vi "main.vi"() -> ()   [LabVIEW 2014]
uses:
  mainVIs/wczytajDaneDoRuchuVIs/Akcje_wczytywania_danych_do_ruchu.ctl
  mainVIs/wykonajRuchVIs/parametryKomorVIs/WyborKomory.ctl
  mainVIs/AkcjaGFV.ctl
  mainVIs/Stan_glowny.ctl
  <vilib>/MakerHub/LINX/Public/Utilities/Open Local.vi
  <vilib>/MakerHub/LINX/LMH-LINX.lvlib
panel:
  out "Pomiar":bool
  out "Czujnik":bool
  in  "Stop":bool
  in  "Dӣ":bool
  in  "GÓRA":bool
  in  "LEWO":bool
  in  "PRAWO":bool
  in  "Praca ręczna":bool
  in  "Start":bool
  out "Działanie ramienia":bool
  out "Góra":bool
  out "Dół":bool
  out "Prawo":bool
  out "Lewo":bool
  # "Praca ręczna"
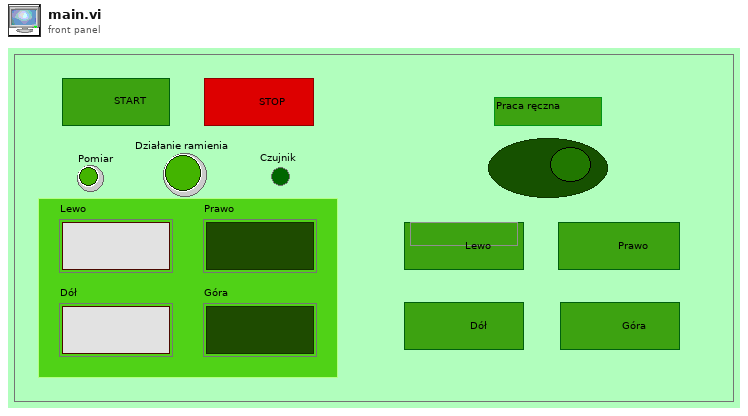
[diagram p1: front panel]
types:
  T1 = typedef "WyborKomory.ctl" = enum16{"NADAWCZA", "ODBIORCZA"}
  T2 = typedef "Akcje_wczytywania_danych_do_ruchu.ctl" = enum16{"Init", "Reset ramienia", "Przygotuj listę", "Sprawdź", "Koniec"}
  T3 = typedef "Stan_glowny.ctl" = enum16{"Oczekiwanie", "Init", "Działanie"}
  T4 = typedef "AkcjaGFV.ctl" = enum16{"Czytaj", "Zapisz", "Reset"}
  T5 = typedef "LMH-LINX.lvlib/LINX Ref.ctl" = cluster{"IO":T6, "Interface":T7, "LINX Device Config":T8}
  T6 = typedef "LMH-LINX.lvlib/Platform.ctl" = enum16{"Remote", "Local"}
  T7 = typedef "LMH-LINX.lvlib/Interface.ctl" = enum16{"Serial", "TCP"}
  T8 = typedef "LMH-LINX.lvlib/Device.lvlib/LINX Device Config.ctl" = cluster{"Interface":T7, "COM Port":refnum<visa-resource-name>, "TCP Configuration":T9, "Device Family":u8, "Device ID":u8, "Device Name":string, "TCP Ref":refnum<k5>, "Channels":T10}
  T9 = typedef "LMH-LINX.lvlib/Device.lvlib/TCP Config.ctl" = cluster{"IP Address":string, "Port":u16}
  T10 = typedef "LMH-LINX.lvlib/Channels.ctl" = cluster{"DI":u8[], "DO":u8[], "AI":u8[], "AO":u8[], "PWM":u8[], "QE":u8[], "UART":u8[], "I2C 2":u8[], "SPI":u8[], "CAN":u8[], "Servo":u8[], "AI Ref (V)":dbl, "AI Resolution (Bits)":u8, "AO Ref (V)":dbl, "AO Resolution (Bits)":u8}
  T11 = typedef "Przyciski_zbior.ctl" = cluster{"LEWO":bool, "PRAWO":bool, "GÓRA":bool, "Dӣ":bool, "Stop":bool, "Start":bool, "Praca ręczna":bool}
  T12 = typedef "Diody_zbior.ctl" = cluster{"Lewo":bool, "Prawo":bool, "Góra":bool, "Dół":bool, "Działanie":bool, "Czujnik":bool, "Pomiar":bool}
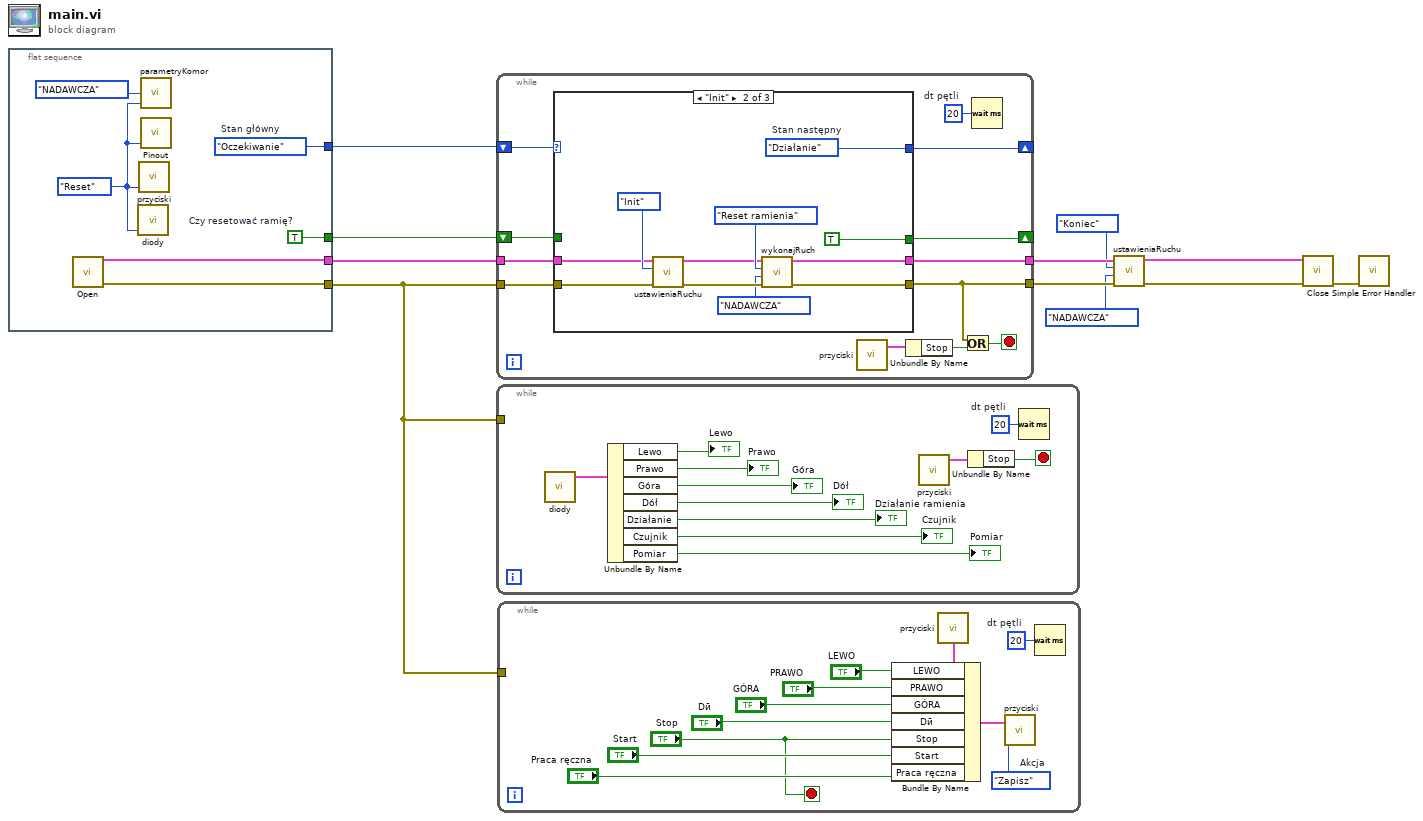
[diagram p0: block diagram]
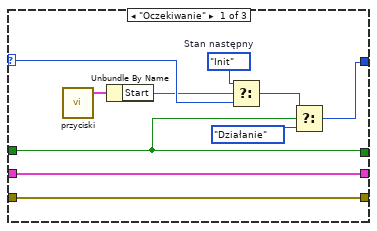
[diagram p2: hidden frame]
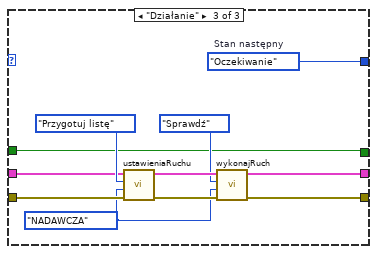
[diagram p3: hidden frame]
diagram:
  n1 = flat-sequence {
    tunnel: [w15] -> w9
    tunnel: [w16] -> w11
    tunnel: [w17] -> w8
    tunnel: [w14] -> w4
    frame #0 {
      w14 = TRUE  # Czy resetować ramię?
      w17 = Stan_glowny."Oczekiwanie"  # Stan główny
      w12 = AkcjaGFV."Reset" ("Akcja")
      n2 = call-poly <vilib>:"Open.vi"() -> ("Error Out"=w15:errorcluster, "LINX Resource"=w16:T5)  [unwired: 9 in, 1 out]
      n3 = call "diody.vi"("Akcja"=w12) -> ()  [unwired: 4 in, 1 out]
      n4 = call "przyciski.vi"("Akcja"=w12) -> ()  [unwired: 4 in, 1 out]
      n5 = call "parametryKomor.vi"("Akcja"=w12, "Wybór komory"=WyborKomory."NADAWCZA" ("Wybór_ramienia")) -> ()  [unwired: 3 in, 1 out]
      n6 = call "Pinout.vi"("Akcja"=w12) -> ()  [unwired: 4 in, 1 out]
    }
  }
  n7 = while {
    shift-right: [w25] -> _
    shift-left: w8 -> [w29]
    tunnel: w11 -> [w28]
    tunnel: w9 -> [w27]
    tunnel: [w26] -> w7
    tunnel: [w20] -> w6
    shift-right: [w18] -> _
    shift-left: w4 -> [w19]
    stop <- w22 stop-if-true
    w24 = u32 20  # dt pętli
    n8 = case shown="\"Init\"" w29 {
      selector: w29 -> [w37 _ _]
      tunnel: w28 -> [w38 w43 w55]
      tunnel: w27 -> [w39 w42 w54]
      tunnel: [w38 w50 w58] -> w26
      tunnel: [w39 w49 w57] -> w20
      tunnel: [w30 w48 w56] -> w25
      tunnel: w19 -> [w33 _ w52]
      tunnel: [w33 TRUE w52] -> w18
      frame "Oczekiwanie" {
        w36 = Stan_glowny."Init"  # Stan następny
        n9 = call "przyciski.vi"() -> ("Wyjście"=w35:T11)  [unwired: 5 in]
        n10 = Unbundle By Name(w35) -> ("Start"=w34:bool)
        n11 = Select(t=w36, s=w34, f=w37) -> (s? t:f=w32:T3)
        n12 = Select(t=w32, s=w33, f=Stan_glowny."Działanie") -> (s? t:f=w30:T3)
      }
      frame "Init" {
        w48 = Stan_glowny."Działanie"  # Stan następny
        n13 = call "ustawieniaRuchu.vi"("error in"=w42, "Rodzaj akcji"=Akcje_wczytywania_danych_do_ruchu."Init" ("Akcja"), "LINX Resource in"=w43) -> ("error out"=w44:errorcluster, "LINX Resource out"=w45:T5)  [unwired: 5 in]
        n14 = call "wykonajRuch.vi"("error in (no error)"=w44, "Wybór komory"=WyborKomory."NADAWCZA", "Akcja"=Akcje_wczytywania_danych_do_ruchu."Reset ramienia", "LINX Resource in"=w45) -> ("error out"=w49:errorcluster, "LINX Resource out"=w50:T5)  [unwired: 6 in]
      }
      frame "Działanie" {
        w51 = WyborKomory."NADAWCZA" ("Wybór komory")
        w56 = Stan_glowny."Oczekiwanie"  # Stan następny
        n15 = call "ustawieniaRuchu.vi"("error in"=w54, "Wybór komory"=w51, "Rodzaj akcji"=Akcje_wczytywania_danych_do_ruchu."Przygotuj listę" ("Akcja"), "LINX Resource in"=w55) -> ("error out"=w61:errorcluster, "LINX Resource out"=w60:T5)  [unwired: 4 in]
        n16 = call "wykonajRuch.vi"("error in (no error)"=w61, "Wybór komory"=w51, "Akcja"=Akcje_wczytywania_danych_do_ruchu."Sprawdź", "LINX Resource in"=w60) -> ("error out"=w57:errorcluster, "LINX Resource out"=w58:T5)  [unwired: 6 in]
      }
    }
    n17 = call "przyciski.vi"() -> ("Wyjście"=w23:T11)  [unwired: 5 in]
    n18 = Unbundle By Name(w23) -> ("Stop"=w21:bool)
    n19 = Or(x=w20, y=w21) -> (x .or. y?=w22:bool)
    n20 = Wait (ms)(milliseconds to wait=w24) -> ()  [unwired: 1 out]
  }
  n21 = while {
    tunnel: w9 -> [_]
    stop <- w64 stop-if-true
    w72 = u32 20  # dt pętli
    n22 = call "diody.vi"() -> ("Wyjście"=w71:T12)  [unwired: 5 in]
    n23 = Unbundle By Name(w71) -> ("Lewo"=→"Lewo":bool, "Prawo"=→"Prawo":bool, "Góra"=→"Góra":bool, "Dół"=→"Dół":bool, "Działanie"=→"Działanie ramienia":bool, "Czujnik"=→"Czujnik":bool, "Pomiar"=→"Pomiar":bool)
    n24 = call "przyciski.vi"() -> ("Wyjście"=w65:T11)  [unwired: 5 in]
    n25 = Unbundle By Name(w65) -> ("Stop"=w64:bool)
    n26 = Wait (ms)(milliseconds to wait=w72) -> ()  [unwired: 1 out]
  }
  n27 = while {
    tunnel: w9 -> [_]
    stop <- "Stop" stop-if-true
    w73 = AkcjaGFV."Zapisz"  # Akcja
    w83 = u32 20  # dt pętli
    n28 = call "przyciski.vi"() -> ("Wyjście"=w82:T11)  [unwired: 5 in]
    n29 = Bundle By Name(cluster=w82, "LEWO"="LEWO", "PRAWO"="PRAWO", "GÓRA"="GÓRA", "Dӣ"="Dӣ", "Stop"="Stop", "Start"="Start", "Praca ręczna"="Praca ręczna") -> (w75:T11)
    n30 = call "przyciski.vi"("Akcja"=w73, "Wejście"=w75) -> ()  [unwired: 3 in, 1 out]
    n31 = Wait (ms)(milliseconds to wait=w83) -> ()  [unwired: 1 out]
  }
  n32 = call "ustawieniaRuchu.vi"("error in"=w6, "Wybór komory"=WyborKomory."NADAWCZA", "Rodzaj akcji"=Akcje_wczytywania_danych_do_ruchu."Koniec", "LINX Resource in"=w7) -> ("error out"=w2:errorcluster, "LINX Resource out"=w3:T5)  [unwired: 4 in]
  n33 = call <vilib>:"Close.vi"("Error In"=w2, "LINX Resource"=w3) -> ("Error Out"=w10:errorcluster)  [unwired: 9 in]
  n34 = call <vilib>:"Simple Error Handler.vi"("error in (no error)"=w10) -> ()  [unwired: 4 in, 5 out]
